vi "Stop Rx With Report.vi"(0 "_hResourceContext":u32, 1 "secErrPkt":i32, 5 "totalPkt":i32, 7 "goodPackets":i32, 9 "crcErrPkt":i32, 11 "error in (no error)":errorcluster, 12 "rssi":i32) -> (3 "secErrPkt out":i32, 4 "_hResourceContext out":u32, 6 "totalPkt out":i32, 8 "goodPackets out":i32, 10 "crcErrPkt out":i32, 14 "rssi out":i32, 15 "error out":errorcluster)   [LabVIEW 2013, in "QCAWLAN_DLL.lvlib"]
doc: "QCA_DLL_Export void StopRxWithReport(HANDLE _hResourceContext, int* totalPkt, int* goodPackets, int* crcErrPkt, int* secErrPkt, int* rssi);"
uses:
  QCAWLAN_DLL.lvlib
  QCAWLAN_DLL.dll
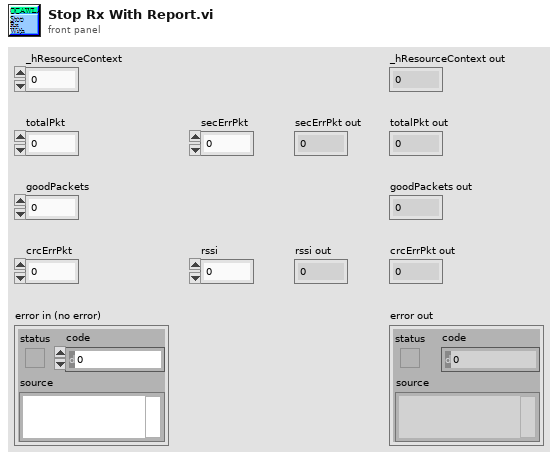
[diagram p1: front panel]
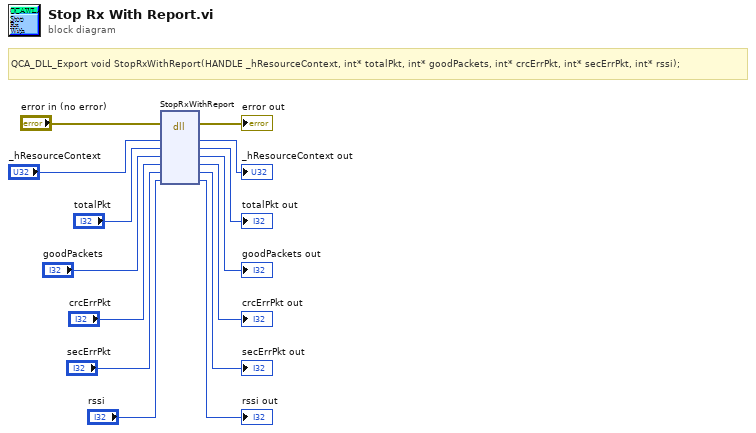
[diagram p0: block diagram]
diagram:
  # "QCA_DLL_Export void StopRxWithReport(HANDLE _hResourceContext, int* totalPkt, int* goodPackets, int* crcErrPkt, int* secErrPkt, int* rssi);"
  n1 = dll-call lib="C:/Connectivity Client - MIMO/PlugIn/QCAWLAN_DLL.*" fn="StopRxWithReport"(error in="error in (no error)", "_hResourceContext"="_hResourceContext", "totalPkt"="totalPkt", "goodPackets"="goodPackets", "crcErrPkt"="crcErrPkt", "secErrPkt"="secErrPkt", "rssi"="rssi") -> (error out=→"error out":errorcluster, "_hResourceContext"=→"_hResourceContext out":u32, "totalPkt"=→"totalPkt out":i32, "goodPackets"=→"goodPackets out":i32, "crcErrPkt"=→"crcErrPkt out":i32, "secErrPkt"=→"secErrPkt out":i32, "rssi"=→"rssi out":i32)  [unwired: 3 in, 1 out]
